vi "PM100D_Meas.vi"(4 "error in":errorcluster, 5 "Timeout":i32=10, 6 "ConfPara":string, 7 "VISA Out":refnum<visa-resource-name>) -> (0 "error out":errorcluster, 1 "Boolean":bool, 2 "ReadValue":string, 3 "dup VISA session":refnum<visa-resource-name>)   [LabVIEW 2011]
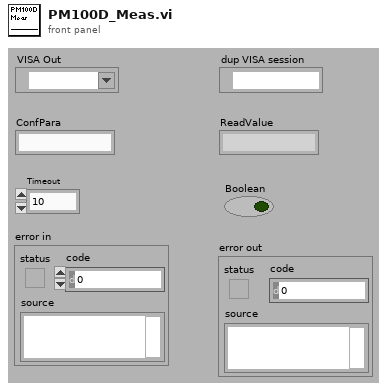
[diagram p1: front panel]
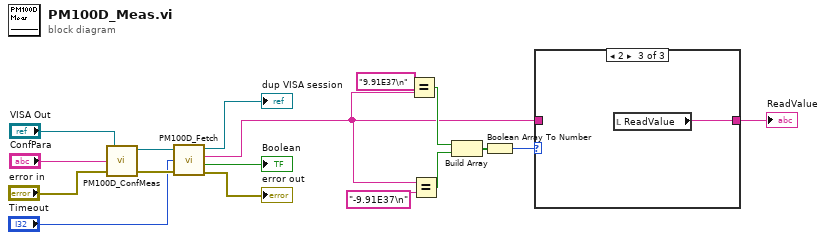
[diagram p0: block diagram]
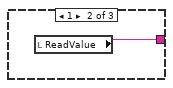
[diagram p3: hidden frame]
diagram:
  n1 = call "PM100D_ConfMeas.vi"("error in"="error in", "Conf:"="ConfPara", "VISA In"="VISA Out") -> ("error out"=w14:errorcluster, "dup VISA session"=w11:refnum<visa-resource-name>)
  n2 = call "PM100D_Fetch.vi"("VISA In"=w11, "Timeout"="Timeout", "error in"=w14) -> ("VISA Out"=→"dup VISA session":refnum<visa-resource-name>, "ReadValue"=w2:string, "Boolean"=→"Boolean":bool, "error out"=→"error out":errorcluster)
  n3 = Equal?(x="9.91E37\n", y=w2) -> (x = y?=w4:bool)
  n4 = Equal?(x=w2, y="-9.91E37\n") -> (x = y?=w5:bool)
  n5 = Build Array(w4, w5) -> (w6:bool[])
  n6 = Boolean Array To Number(Boolean array=w6) -> (number=w3:u32)
  n7 = case shown="2" w3 {
    tunnel: w2 -> [w18 _ _]
    tunnel: [w18 w19 w20] -> w1
    frame 0, Default {
    }
    frame 1 {
      n8 = local read "ReadValue"() -> (w19:string)
    }
    frame 2 {
      n9 = local read "ReadValue"() -> (w20:string)
    }
  }
  "ReadValue" <- w1
